vi "ServerCertification.vi"(3 "xml content":string="<?xml version=\"1.0\" encoding=\"utf-8\"?><opcua_server><name>Faraday Cup Control System</name><port>4845</port><policy>basic128rsa125</policy><serverCertification></serverCertification><trustedClientCertifications>  <certification></certification></trustedClientCertifications><structure>    <folder name=\"System\">        <item name=\"Server URL\" ,access=\"read/write\" datatype=\"string\" initialValue=\"\" description=\"Server URL.\"></item>    </folder>    <folder name=\"Motion\">        <folder name=\"Contorl\">            <item name=\"Power Enable\" access=\"read/write\" datatype=\"boolean\" initialValue=\"FALSE\" description=\"Enable the motion power.\"></item>            <item name=\"Start Move\" access=\"read/write\" datatype=\"boolean\" initialValue=\"FALSE\" description=\"Start to move.\"></item>            <item name=\"Stop Move\" access=\"read/write\" datatype=\"boolean\" initialValue=\"FALSE\" description=\"Stop the movement.\"></item>            <item name=\"Find Home\" access=\"read/write\" datatype=\"boolean\" initialValue=\"FALSE\" description=\"Start to find home.\"></item>        </folder>        <folder name=\"Status\">            <item name=\"FWD Limit\" access=\"read\" datatype=\"boolean\" initialValue=\"FALSE\" description=\"Show the status of fwd limit.\"></item>            <item name=\"REV Limit\" access=\"read\" datatype=\"boolean\" initialValue=\"FALSE\" description=\"Show the status of rev limit.\"></item>            <item name=\"STO\" access=\"read\" datatype=\"boolean\" initialValue=\"FALSE\" description=\"Show the status of STO.\"></item>            <item name=\"Move Complete\" access=\"read\" datatype=\"boolean\" initialValue=\"FALSE\" description=\"Show the status of movement.\"></item>            <item name=\"Find Home Complete\" access=\"read\" datatype=\"boolean\" initialValue=\"FALSE\" description=\"show the status of finding home.\"></item>            <item name=\"E Ruler\" access=\"read\" datatype=\"double\" initialValue=\"0\" description=\"Show the Eruler position.\"></item>        </folder>        <folder name=\"Last Error\">            <item name=\"acknowledge\" access=\"read/write\" datatype=\"boolean\" initialValue=\"FALSE\" description=\"Acknowledge last error.\"></item>            <item name=\"code\" access=\"read\" datatype=\"int32\" initialValue=\"0\" description=\"Show the code of last error.\"></item>            <item name=\"info\" access=\"read\" datatype=\"int32\" initialValue=\"0\" description=\"Show the info of last error.\"></item>        </folder>    </folder>    <folder name=\"DAQ\">        <item name=\"Measurement Range\" access=\"read/write\" datatype=\"int16\" initialValue=\"100\" description=\"Measurement range.\"></item>        <item name=\"Intensity\" access=\"read\" datatype=\"double\" initialValue=\"100\" description=\"Intensity Value.\"></item>        <item name=\"Save file?\" access=\"read/write\" datatype=\"boolean\" initialValue=\"FALSE\" description=\"Enable saving file.\"></item>        <item name=\"File Path\" access=\"read/write\" datatype=\"string\" initialValue=\"\" description=\"Local path of saved file.\"></item>    </folder></structure></opcua_server>") -> (0 "path":path, 1 "xml content(dup)":string)   [LabVIEW 2014, in "OPCUA XML.lvlib"]
uses:
  OPCUA XML.lvlib
panel:
  out "result string":string
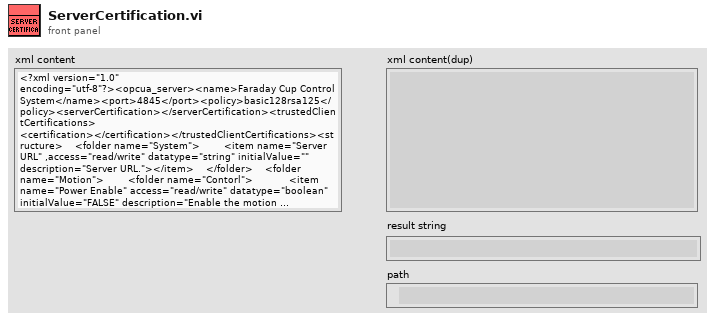
[diagram p1: front panel]
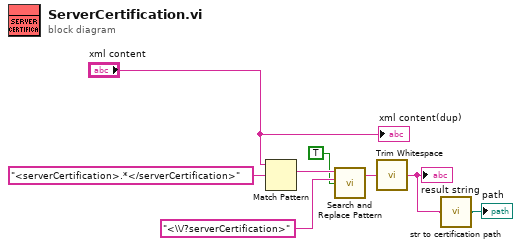
[diagram p0: block diagram]
diagram:
  n1 = Match Pattern(string="xml content", regular expression="<serverCertification>.*</serverCertification>") -> (match substring=w7:string)  [unwired: 1 in, 3 out]
  n2 = call <vilib>:"Search and Replace Pattern.vi"("string"=w7, "regular expression (\"\")"="<\\/?serverCertification>" ("regular expression"), "replace all? (F)"=TRUE) -> ("result string"=w5:string)  [unwired: 2 in, 1 out]
  n3 = call <vilib>:"Trim Whitespace.vi"("string"=w5) -> ("trimmed string"=w2:string)  [unwired: 1 in]
  "result string" <- w2
  n4 = call "str to certification path.vi"("node text"=w2) -> ("File Path Control"=→"path":path)  [unwired: 4 in]
  "xml content(dup)" <- "xml content"
